vi "Workspace.CustomDevices.Get.vi"(8 "error in (no error)":errorcluster, 10 "CD GUID":string, 11 "Target Node":refnum<k24>) -> (0 "error out":errorcluster, 1 "Custom Device Names":string[](array[string]), 2 "Custom Device Nodes":refnum<k24>[](array[refnum]), 3 "Target Node Out":refnum<k24>)   [LabVIEW 2019, in "Ghost Bus Workspace Shared.lvlib"]
uses:
  Ghost Bus Workspace Shared.lvlib
  NationalInstruments.VeriStand.SystemStorage
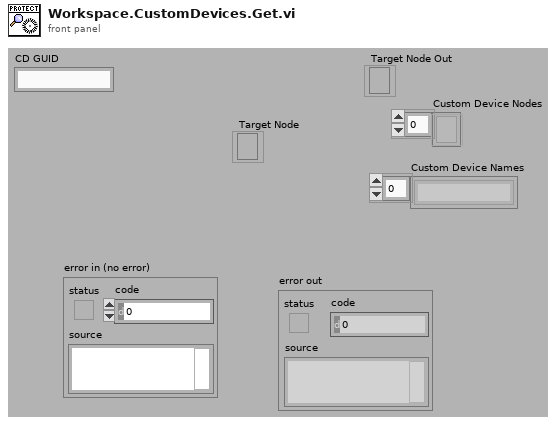
[diagram p1: front panel]
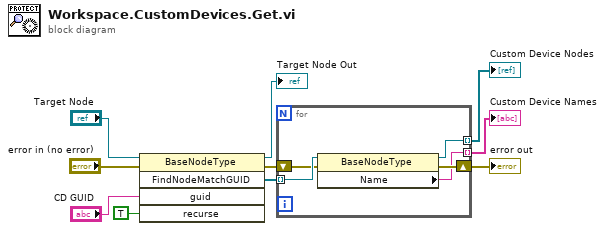
[diagram p0: block diagram]
diagram:
  n1 = invoke class="BaseNodeType" method="FindNodeMatchGUID"(reference="Target Node", error in="error in (no error)", "guid"="CD GUID", "recurse"=TRUE) -> (reference out=→"Target Node Out":refnum<k24>, error out=w9:errorcluster, "FindNodeMatchGUID"=w4:refnum<k24>[])  [unwired: 1 in, 2 out]
  n2 = for {
    tunnel: w4 -> [w15] mode=indexing
    shift-right: [w13] -> w6
    shift-left: w9 -> [w14]
    tunnel: [w12] -> w8 mode=indexing
    tunnel: [w11] -> w7 mode=indexing
    n3 = property class="BaseNodeType"(reference=w15, error in=w14) -> (reference out=w12:refnum<k24>, error out=w13:errorcluster, "Name"=w11:string)
  }
  "error out" <- w6
  "Custom Device Nodes" <- w8
  "Custom Device Names" <- w7
